vi "Waveform-Enumerate Valid Params.vi"(8 "error in (no error)":errorcluster, 11 "Waveform":T17(xcontrol)) -> (0 "error out":errorcluster, 2 "Parameter Names":string[](array[string]))   [LabVIEW 2020]
uses:
  Controls/Waveform XCtl/Waveform XCtl.xctl
  <vilib>/regexp/Match Regular Expression.xnode
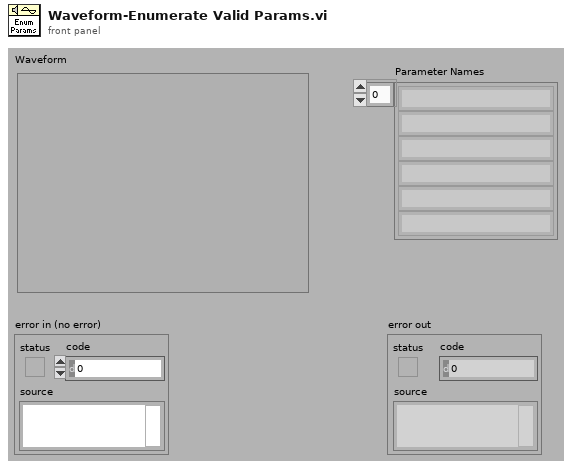
[diagram p1: front panel]
types:
  T1 = typedef "Waveform Enum.ctl" = enum16{"OFF", "Tone", "Noise", "Pulse Train", "File", "FM Sweep", "Chirp Train", "Complex Tone", "FM Tone", "Moving Ripple"}
  T2 = typedef "Tone Params.ctl" = cluster{"Frequency (kHz)":dbl, "Last Freq":dbl, "Last Phase":dbl}
  T3 = typedef "Pulse Train Params.ctl" = cluster{"Pulse width (us)":dbl, "Pulse rate (Hz)":dbl, "Gap (ms)":dbl, "Polarity":T4, "PT State":T5, "Asynch":bool}
  T4 = typedef "Pulse Polarity.ctl" = enum16{"POS", "NEG", "POS-NEG", "NEG-POS"}
  T5 = typedef "PT-Continuous State.ctl" = cluster{"Template":dbl[], "Nperiod":i32, "Index":i32, "Pulse Rate (Hz)":dbl, "Phase (cycles)":dbl, "Noff":i32}
  T6 = typedef "Noise Params.ctl" = cluster{"InvFilt":bool, "Noise":dbl[], "CurPt":i32, "Aweight":bool, "Seed":i32, "afile":path}
  T7 = typedef "StimFile-Params.ctl" = cluster{"Filename":path, "Signal":dbl[], "Channel":i32, "stream":bool, "offset":i32, "nreps":i32, "loops":i32, "Randomize":bool, "order":i32[], "Seed":i32, "Tokens":i32}
  T8 = typedef "FM Sweep Params.ctl" = cluster{"Rate (oct/s)":dbl, "Fmin (Hz)":dbl, "Fmax (Hz)":dbl, "Ramp (ms)":dbl, "Linear":bool}
  T9 = typedef "Chirp Train.ctl" = cluster{"Params":T10, "Data":cluster{"WF":dbl[]}}
  T10 = typedef "Chirp Train Params.ctl" = cluster{"Fmin (kHz)":dbl, "Fmax (kHz)":dbl, "Compensate":bool, "Duration (ms)":dbl}
  T11 = typedef "CT-Params.ctl" = cluster{"F0 (Hz)":dbl, "Band":cluster{"Flow (Hz)":dbl, "Fhigh (Hz)":dbl}, "Phase":T12, "Min F0 (Hz)":dbl, "Max F0 (Hz)":dbl, "ContinRandPhase":bool, "Max peak factor":dbl, "Max mod depth":dbl, "MinHarmNum":i32, "MaxHarmNum":i32, "Level Mode":enum16{"per component", "overall rms"}, "% jitter":dbl}
  T12 = typedef "CT-Phase Enum.ctl" = enum16{"Cosine", "Random", "Alternating"}
  T13 = typedef "CT-Runtime Data.ctl" = cluster{"Ncomp":i32, "MinHarm":i32, "Phase":dbl[], "Amplitude":dbl[], "Npts/frame":i32, "Last F0":dbl, "Fmin":dbl, "Fmax":dbl, "Lslope":dbl, "randphase":bool, "overall rms":bool, "fmult":dbl[], "jittered":bool}
  T14 = typedef "Moving Ripple.ctl" = cluster{"Params":T15, "Data":T16}
  T15 = typedef "Moving Ripple.Params.ctl" = cluster{"Fmin":dbl, "Fmax":dbl, "Density":dbl, "Velocity":dbl, "Depth":dbl, "Phase":dbl, "Comp/oct":i32}
  T16 = typedef "Moving Ripple.Data.ctl" = cluster{"Freq":dbl[], "A":dbl[], "phase":dbl[], "Phase":dbl}
  T17 = cluster{"Type":T1, "Tone":T2, "Pulse Train":T3, "Noise":T6, "File":T7, "FMSweep":T8, "Chirp Train":T9, "Complex Tone":cluster{"Params":T11, "Data":T13}, "Moving Ripple":T14}
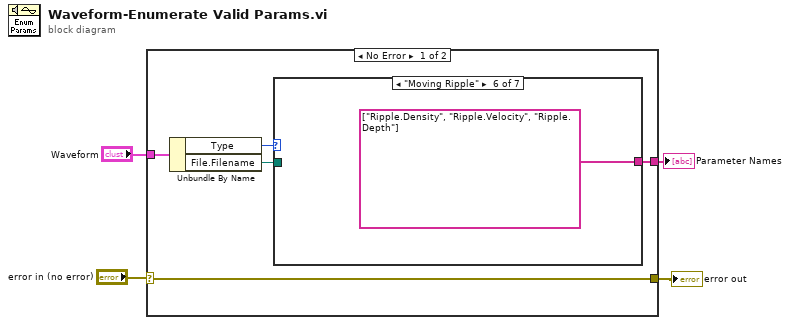
[diagram p0: block diagram]
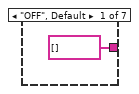
[diagram p2: hidden frame]
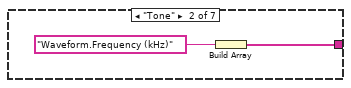
[diagram p3: hidden frame]
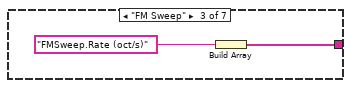
[diagram p4: hidden frame]
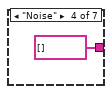
[diagram p5: hidden frame]
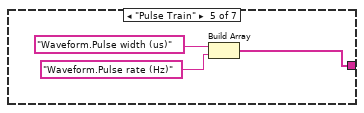
[diagram p6: hidden frame]
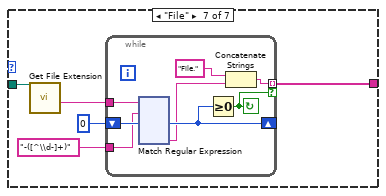
[diagram p7: hidden frame]
diagram:
  n1 = case shown="No Error" "error in (no error)" {
    selector: "error in (no error)" -> [w6 w149]
    tunnel: "Waveform" -> [w8 _]
    tunnel: [w7 _] -> w3
    tunnel: [w6 w149] -> w1
    frame No Error {
      n2 = Unbundle By Name(w8) -> ("Type"=w9:T1, "File.Filename"=w5:path)
      n3 = case shown="\"Moving Ripple\"" w9 {
        tunnel: [string[] [] w11 w13 string[] [] w16 string[] ["Ripple.Density", "Ripple.Velocity", "Ripple.Depth"] w20] -> w7
        tunnel: w5 -> [_ _ _ _ _ _ w24]
        frame "OFF", Default {
        }
        frame "Tone" {
          n4 = Build Array("Waveform.Frequency (kHz)" ("String")) -> (w11:string[])
        }
        frame "FM Sweep" {
          n5 = Build Array("FMSweep.Rate (oct/s)" ("String")) -> (w13:string[])
        }
        frame "Noise" {
        }
        frame "Pulse Train" {
          n6 = Build Array("Waveform.Pulse width (us)" ("String"), "Waveform.Pulse rate (Hz)" ("String")) -> (w16:string[])
        }
        frame "Moving Ripple" {
        }
        frame "File" {
          n7 = call <vilib>:"Get File Extension.vi"("file"=w24) -> ("filename without extension"=w23:string)  [unwired: 6 in, 4 out]
          n8 = while {
            tunnel: w23 -> [w32]
            shift-right: [w29] -> _
            shift-left: 0 -> [w31]
            tunnel: "-([^\\d-]+)" -> [w30]
            tunnel: [w26] -> w20 mode=indexing if=w27
            stop <- w27 continue-if-true
            n9 = xnode "Match Regular Expression"("input string"=w32, "regular expression"=w30, "offset (0)"=w31) -> ("offset past match"=w29:i32, "submatch 1"=w28:string)  [unwired: 3 in, 4 out]
            n10 = Greater Or Equal To 0?(x=w29) -> (x >= 0?=w27:bool)
            n11 = Concatenate Strings("File." ("string"), w28) -> (w26:string)
          }
        }
      }
    }
    frame Error {
    }
  }
  "error out" <- w1
  "Parameter Names" <- w3
